vi "flattenLengthToXML.vi"   [LabVIEW 2012, in "UnitsAndXML.lvlib"]
doc: "Generates an XML string for <B>length</B> in the unit specified in <B>lengthUnitInXML</B>. Connect <B>length</B> and <B>lengthAgain</B> to the same source. The VI uses <B>lengthAgain</B> to obtain the data name."
uses:
  <userlib>/Common/UnitsAndXML/UnitsAndXML.lvlib
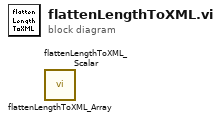
[diagram p0: block diagram]
diagram:
  n1 = call <userlib>:"flattenLengthToXML_Array.vi"() -> ()  [unwired: 10 in, 2 out]
  n2 = call <userlib>:"flattenLengthToXML_Scalar.vi"() -> ()  [unwired: 10 in, 2 out]
